vi "Drive Turn degree.vi"(11 "Degrees":dbl) -> ()   [LabVIEW 2017]
panel:
  in  "stop":bool
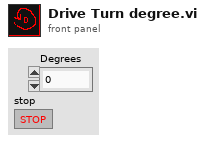
[diagram p1: front panel]
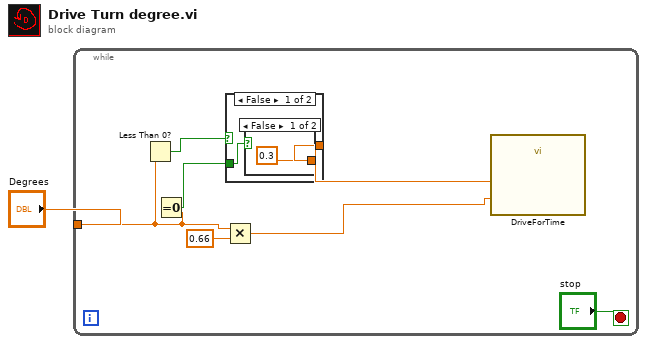
[diagram p0: block diagram]
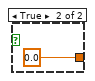
[diagram p2: hidden frame]
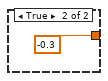
[diagram p3: hidden frame]
diagram:
  n1 = while {
    tunnel: "Degrees" -> [w4]
    stop <- "stop" stop-if-true
    n2 = Less Than 0?(x=w4) -> (x < 0?=w7:bool)
    n3 = Equal To 0?(x=w4) -> (x = 0?=w8:bool)
    n4 = Multiply(x=w4, y=0.66) -> (x*y=w3:dbl)
    n5 = case shown="False" w7 {
      tunnel: [w9 -0.3] -> w6
      tunnel: w8 -> [w10 _]
      frame False {
        n6 = case shown="False" w10 {
          tunnel: [0.3 0.0] -> w9
          frame False {
          }
          frame True {
          }
        }
      }
      frame True {
      }
    }
    n7 = call "DriveForTime.vi"("Time(s)"=w3, "Rotation"=w6) -> ()  [unwired: 10 in]
  }
